vi "StringToGs.vi"(7 "String":string="-0194") -> (8 "Gs":dbl)   [LabVIEW 2014]
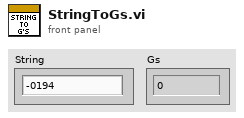
[diagram p1: front panel]
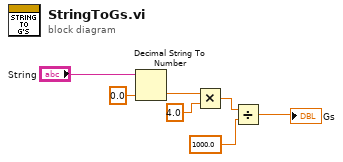
[diagram p0: block diagram]
diagram:
  n1 = Decimal String To Number(string="String", default (0L)=0.0 ("default (0 I32)")) -> (number=w5:dbl)  [unwired: 1 in, 1 out]
  n2 = Multiply(x=w5, y=4.0) -> (x*y=w3:dbl)
  n3 = Divide(x=w3, y=1000.0) -> (x/y=→"Gs":dbl)
